vi "STAT2 decode Analog data from Solonoid Node.vi"(9 "Temperature base conversion factor":u16=128, 10 "Solonoid":T1 {"valve status" format="%02x"; "sys register" format="%04x"}) -> (2 "Node Analog value":dbl[](array[numeric]), 3 "Temperature":dbl)   [LabVIEW 2011]
uses:
  LEINmaster/Nodes/solonoid stat2.ctl
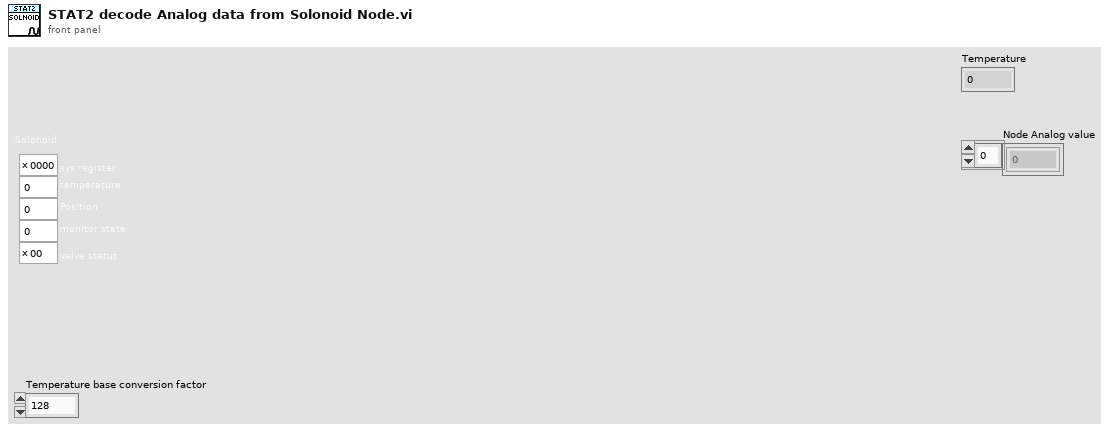
[diagram p1: front panel]
types:
  T1 = typedef "solonoid stat2.ctl" = cluster{"sys register":u16, "temperature":u16, "Position":i16, "monitor state":u8, "valve status":u8}
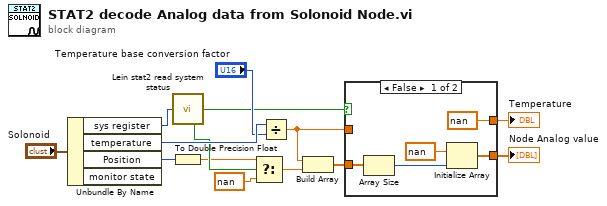
[diagram p0: block diagram]
diagram:
  n1 = Unbundle By Name("Solonoid") -> ("sys register"=w9:u16, "temperature"=w14:u16, "Position"=w5:i16)  [unwired: 1 out]
  n2 = call "Lein stat2 read system status.vi"("sys register"=w9) -> ("Connected"=w12:bool, "User bit"=w3:bool)  [unwired: 7 in, 6 out]
  n3 = To Double Precision Float(number=w5) -> (double precision float=w1:dbl)
  n4 = Select(t=w1, s=w3, f=nan) -> (s? t:f=w2:dbl)
  n5 = Divide(x=w14, y="Temperature base conversion factor") -> (x/y=w8:dbl)
  n6 = Build Array(w8, w2) -> (w11:dbl[])
  n7 = case shown="False" w12 {
    tunnel: [w16 w21] -> w10
    tunnel: w11 -> [w19 w21]
    tunnel: [nan ("element") w20] -> w7
    tunnel: w8 -> [_ w20]
    frame False {
      n8 = Array Size(array=w19) -> (size(s)=w18:i32)
      n9 = Initialize Array(nan ("element"), w18) -> (w16:dbl[])
    }
    frame True {
    }
  }
  "Node Analog value" <- w10
  "Temperature" <- w7
